vi "SetName Anchor.vi"(0 "Leading":sgl=1.5, 1 "Text zone (points)":cluster{"widht":sgl, "height":sgl}={"widht"=612.0, "height"=792.0}, 5 "Text":string, 7 "Image to Add refnum [ ]":T3, 9 "Font refnum":refnum<k24>, 11 "error in (no error)":errorcluster, 12 "Type and run direction":T1=enum."ASCII", 13 "Paragraph indentation (points)":T2) -> (4 "Leading OUT":sgl=1.5, 6 "Anchor":refnum<k24>, 15 "error out":errorcluster)   [LabVIEW 2020, in "Exaprom PDF.lvlib"]
doc: "Creates a <B>text hyperlink</B>.\n\nVersion 2.0\nDeveloped by Jean-Marc Simard\nCopyright © 2013, Exaprom Inc.\nAll rights reserved.\nLicense: BSD\n\nWith iTextSharp 4.1.6 (http://itextsharp.sourceforge.net)\nunder Mozilla Public License Version 1.1\n(http://www.mozilla.org/MPL/MPL-1.1.html)"
uses:
  <userlib>/labview-PDF-writer-master/Exaprom PDF.lvlib
  C:/Program Files (x86)/National Instruments/LabVIEW 2020/user.lib/labview-PDF-writer-master/DLL/itextsharp.dll
  DLL/itextsharp.dll
  <userlib>/labview-PDF-writer-master/Controls/General Controls/Image to Add refnum [ ].ctl
  <userlib>/labview-PDF-writer-master/Controls/Text Controls/Paragraph indentation.ctl
  <userlib>/labview-PDF-writer-master/Controls/Text Controls/Unicode/Type and run direction.ctl
  <userlib>/labview-PDF-writer-master/Controls/Text Controls/Phrase or paragraph.ctl
panel:
  # "设置名称"
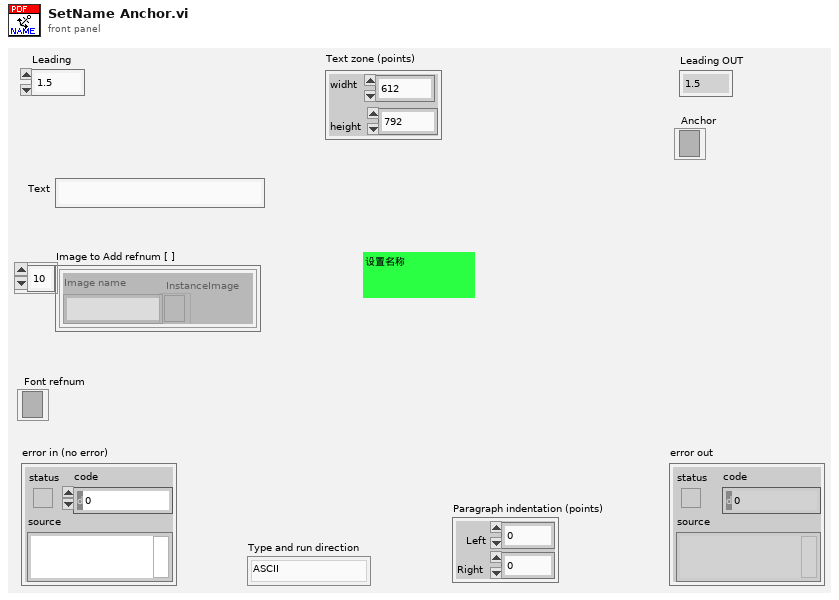
[diagram p1: front panel]
types:
  T1 = typedef "Exaprom PDF.lvlib/Type and run direction.ctl" = enum16{"Select", "ASCII", "UTF-16", "UTF-16 (default)", "UTF-16 (LTR)", "UTF-16 (RTL)"}
  T2 = typedef "Exaprom PDF.lvlib/Paragraph indentation.ctl" = cluster{"Left":sgl, "Right":sgl}
  T3 = typedef "Exaprom PDF.lvlib/Image to Add refnum [ ].ctl" = cluster{"Image name":string, "InstanceImage":refnum<k24>}[]
  T4 = typedef "Exaprom PDF.lvlib/Phrase or paragraph.ctl" = enum16{"Add to Phrase", "Add to Paragraph", "Create Phrase", "Create Paragraph"}
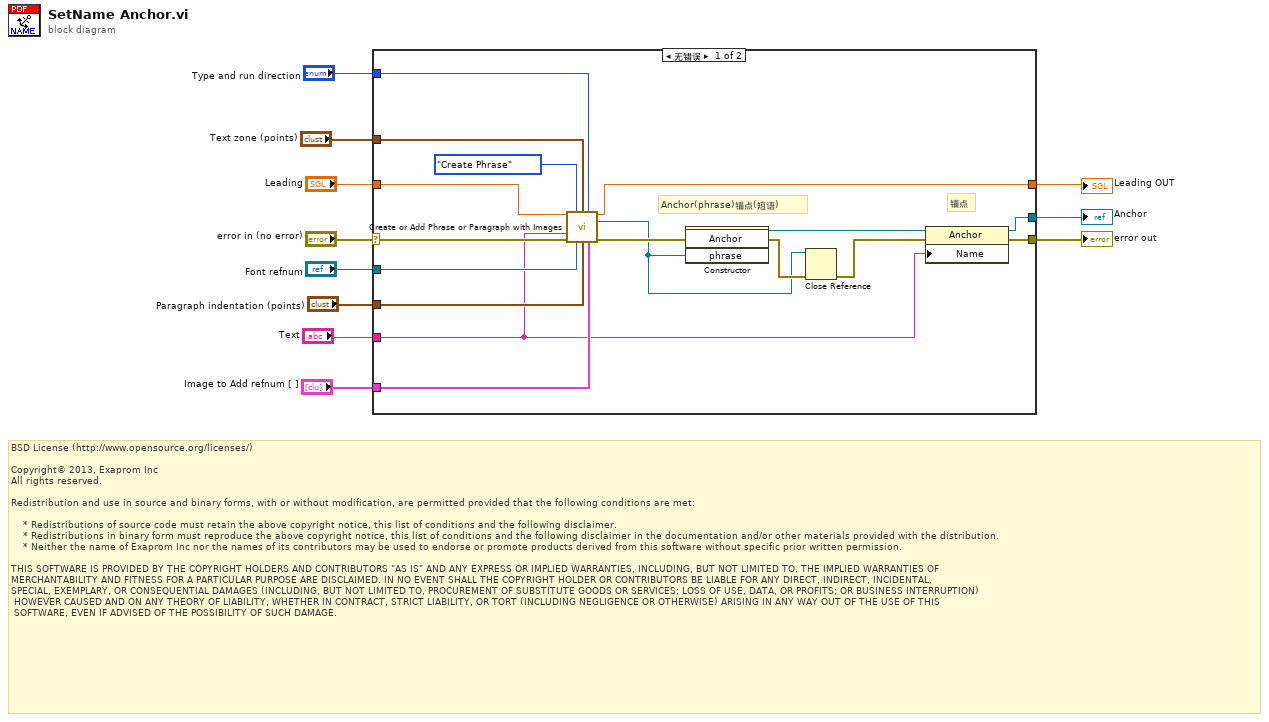
[diagram p0: block diagram]
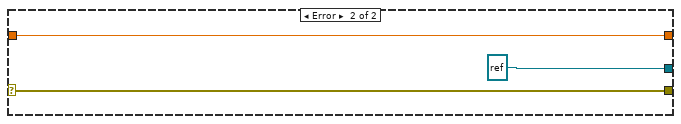
[diagram p2: hidden frame]
diagram:
  # "BSD License (http://www.opensource.org/licenses/)\n\nCopyright© 2013, Exaprom Inc\nAll rights reserved.\n\nRedistribution and use in source and binary forms, with or without modification, are permitted provided that the following conditions are met:\n\n    * Redistributions of source code must retain the above copyright notice, this list of conditions and the following disclaimer.\n    * Redistributions in binary form must reproduce the above copyright notice, this list of conditions and the following disclaimer in the documentation and/or other materials provided with the distribution.\n    * Neither the name of Exaprom Inc nor the names of its contributors may be used to endorse or promote products derived from this software without specific prior written permission.\n\nTHIS SOFTWARE IS PROVIDED BY THE COPYRIGHT HOLDERS AND CONTRIBUTORS \"AS IS\" AND ANY EXPRESS OR IMPLIED WARRANTIES, INCLUDING, BUT NOT LIMITED TO, THE IMPLIED WARRANTIES OF \nMERCHANTABILITY AND FITNESS FOR A PARTICULAR PURPOSE ARE DISCLAIMED. IN NO EVENT SHALL THE COPYRIGHT HOLDER OR CONTRIBUTORS BE LIABLE FOR ANY DIRECT, INDIRECT, INCIDENTAL,\nSPECIAL, EXEMPLARY, OR CONSEQUENTIAL DAMAGES (INCLUDING, BUT NOT LIMITED TO, PROCUREMENT OF SUBSTITUTE GOODS OR SERVICES; LOSS OF USE, DATA, OR PROFITS; OR BUSINESS INTERRUPTION)\n HOWEVER CAUSED AND ON ANY THEORY OF LIABILITY, WHETHER IN CONTRACT, STRICT LIABILITY, OR TORT (INCLUDING NEGLIGENCE OR OTHERWISE) ARISING IN ANY WAY OUT OF THE USE OF THIS\n SOFTWARE, EVEN IF ADVISED OF THE POSSIBILITY OF SUCH DAMAGE."
  n1 = case shown="无错误" "error in (no error)" {
    selector: "error in (no error)" -> [w18 w31]
    tunnel: [w27 w31] -> w11
    tunnel: "Text" -> [w15 _]
    tunnel: [w12 refnum<k24> refnum ("hidden reference")] -> w9
    tunnel: "Leading" -> [w20 w29]
    tunnel: "Font refnum" -> [w26 _]
    tunnel: "Image to Add refnum [ ]" -> [w28 _]
    tunnel: "Text zone (points)" -> [w25 _]
    tunnel: "Paragraph indentation (points)" -> [w21 _]
    tunnel: [w19 w29] -> w4
    tunnel: "Type and run direction" -> [w16 _]
    frame No Error {
      # "Anchor(phrase)锚点(短语)"
      # "锚点"
      n2 = call <userlib>:"Create or Add Phrase or Paragraph with Images.vi"("Leading"=w20, "Phrase or paragraph"=Phrase_or_paragraph."Create Phrase", "Text zone (points)"=w25, "Character type"=w16, "Text"=w15, "error in (no error)"=w18, "Font refnum"=w26, "Paragraph indentation (points)"=w21, "Image to Add refnum [ ]"=w28) -> ("Leading duplicate"=w19:sgl, "Phrase refnum OUT"=w14:refnum<k24>, "error out"=w24:errorcluster)  [unwired: 2 in, 2 out]
      n3 = constructor class="Anchor"(error in=w24, "phrase"=w14) -> (reference out=w13:refnum<k24>, error out=w23:errorcluster)  [unwired: 2 in, 2 out]
      n4 = Close Reference(reference=w14, error in (no error)=w23) -> (error out=w22:errorcluster)
      n5 = property class="Anchor"(reference=w13, error in=w22, "Name"=w15) -> (reference out=w12:refnum<k24>, error out=w27:errorcluster)
    }
    frame Error {
    }
  }
  "error out" <- w11
  "Anchor" <- w9
  "Leading OUT" <- w4
